vi "Write ITX (2D w X&Y).vi"(4 "Commands":string, 6 "Notes":string, 8 "error in":errorcluster, 9 "Wavenames":cluster{"2D":string, "X":string, "Y":string}, 10 "2D, X, Y (Cluster)":T1, 11 "filename":path) -> (0 "error out":errorcluster, 3 "file out":path)   [LabVIEW 2019, in "Data.ITX.lvclass"]
uses:
  Data.ITX.lvclass
panel:
  out "String":string
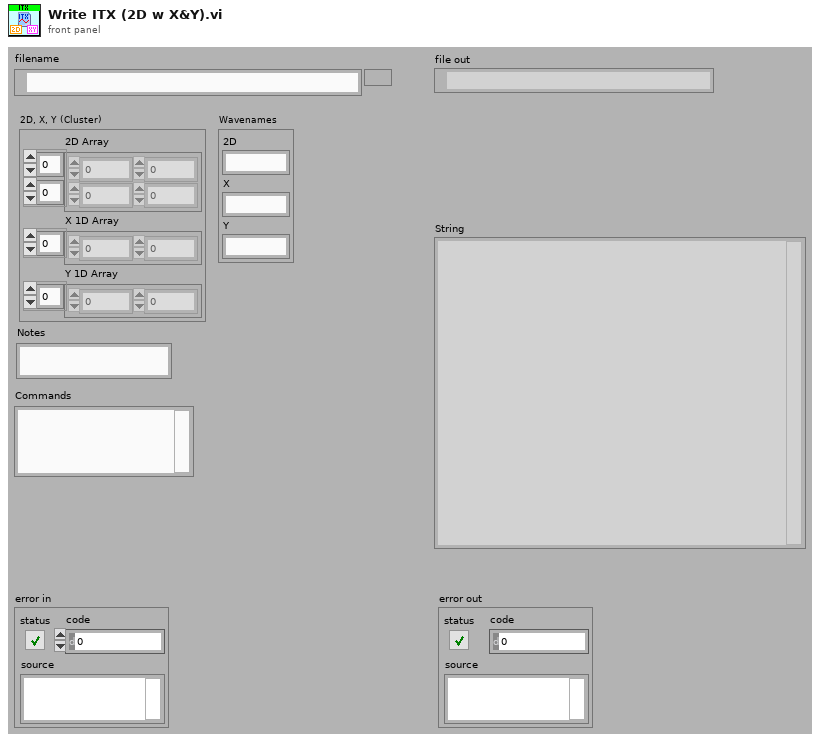
[diagram p1: front panel]
types:
  T1 = cluster{"2D Array":dbl[][], "X 1D Array":dbl[], "Y 1D Array":dbl[]}
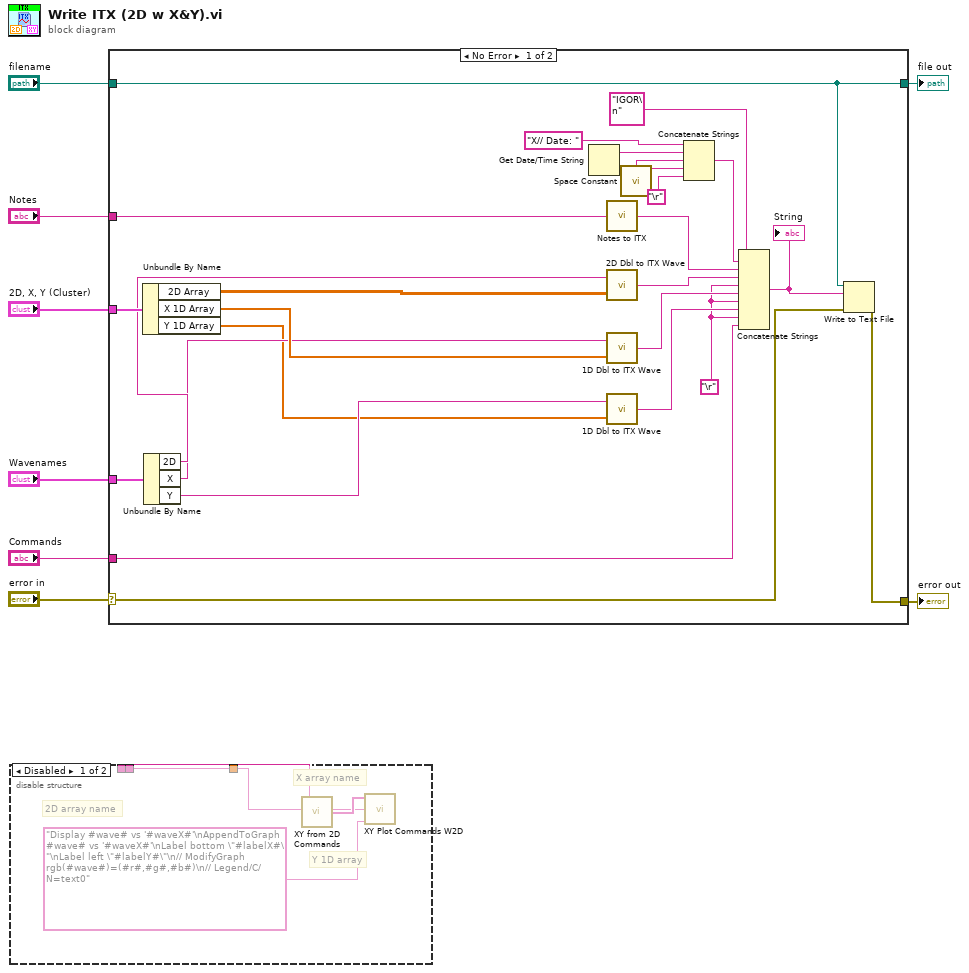
[diagram p0: block diagram]
diagram:
  n1 = disable-structure shown="Disabled" {
    disable-tunnel: _ -> [w13 _]
    disable-tunnel: _ -> [w12 _]
    disable-tunnel: _ -> [w9 _]
    frame Disabled {
      # "Y 1D array"
      # "2D array name"
      # "X array name"
      n2 = call "XY from 2D Commands.vi"("Y 1D Array"=w12, "2D wave"=w13) -> ("wavenames"=w11:string[])
      n3 = call "XY Plot Commands W2D.vi"("wavenames"=w11, "input string"="Display #wave# vs '#waveX#'\nAppendToGraph #wave# vs '#waveX#'\nLabel bottom \"#labelX#\"\nLabel left \"#labelY#\"\n// ModifyGraph rgb(#wave#)=(#r#,#g#,#b#)\n// Legend/C/N=text0", "X wave"=w9) -> ()  [unwired: 2 in, 1 out]
    }
    frame Enabled {
    }
  }
  n4 = case shown="No Error" "error in" {
    selector: "error in" -> [w15 w41]
    tunnel: "Notes" -> [w34 _]
    tunnel: "filename" -> [w24 w40]
    tunnel: "Commands" -> [w14 _]
    tunnel: [w25 w41] -> w4
    tunnel: [w24 w40] -> w3
    tunnel: "2D, X, Y (Cluster)" -> [w23 _]
    tunnel: "Wavenames" -> [w21 _]
    frame No Error {
      w29 = "\r"
      n5 = Unbundle By Name(w23) -> ("2D Array"=w16:dbl[][], "X 1D Array"=w22:dbl[], "Y 1D Array"=w17:dbl[])
      n6 = Unbundle By Name(w21) -> ("2D"=w20:string, "X"=w19:string, "Y"=w18:string)
      n7 = Get Date/Time String() -> (date string=w38:string, time string=w39:string)  [unwired: 3 out]
      n8 = call "Notes to ITX.vi"("Notes"=w34) -> ("ITX Notes"=w30:string)
      n9 = call "2D Dbl to ITX Wave.vi"("2D Array"=w16, "Wavename"=w20) -> ("ITX Wave"=w33:string)
      n10 = call "1D Dbl to ITX Wave.vi"("1D Array"=w22, "Wavename"=w19) -> ("ITX Wave"=w32:string)
      n11 = call "1D Dbl to ITX Wave.vi"("1D Array"=w17, "Wavename"=w18) -> ("ITX Wave"=w31:string)
      n12 = call <vilib>:"Space Constant.vi"() -> ("String"=w27:string)
      n13 = Concatenate Strings("X// Date: " ("format string"), w38, w27, w39, "\r") -> (w37:string)
      n14 = Concatenate Strings("IGOR\n", w37, w30, w33, w29, w32, w29, w31, w29, w14) -> (w28:string)
      "String" <- w28
      n15 = Write to Text File(file (use dialog)=w24, text=w28, error in=w15) -> (error out=w25:errorcluster)  [unwired: 3 out]
    }
    frame Error {
    }
  }
  "file out" <- w3
  "error out" <- w4
